vi "Draw Image to Picture (ARGB with Mask).vi"(7 "Image Draw Offset (Default 0,0)":T2, 8 "error in (no error)":errorcluster, 10 "Greyscale Mask in":T1, 11 "ARGB Image Source in":T3) -> (0 "error out":errorcluster, 3 "Picture":picture)   [LabVIEW 2020, in "image.lvlib"]
doc: "Draw an image to a LabVIEW Picture with Mask Data to allow for the output picture to be concatinated with other LabVIEW Picture Data."
uses:
  image.lvlib
  ARGB Image.ctl
  Image Draw Offset.ctl
  Greyscale Image.ctl
  8cd07b1b-062e-4fe4-9e87-2eb3dc89fe0e.vi
  <vilib>/Utility/error.llb/Error Cluster From Error Code.vi
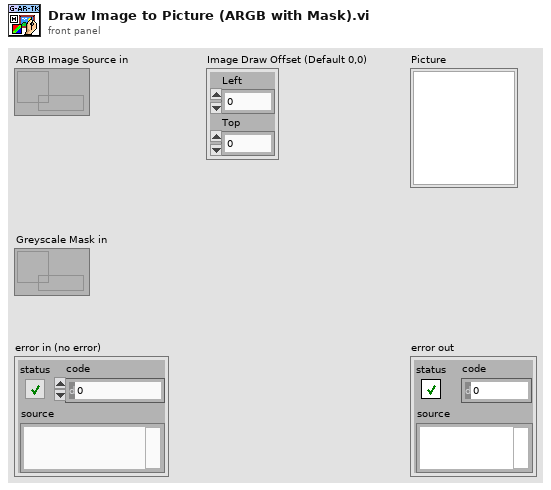
[diagram p1: front panel]
types:
  T1 = typedef "image.lvlib/Greyscale Image.ctl" = refnum<data-value>
  T2 = typedef "image.lvlib/Image Draw Offset.ctl" = cluster{"Left":i16, "Top":i16}
  T3 = typedef "image.lvlib/ARGB Image.ctl" = refnum<data-value>
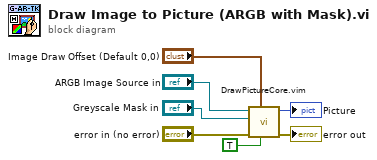
[diagram p0: block diagram]
diagram:
  n1 = call "DrawPictureCore.vim"("HasMask"=TRUE, "Image Draw Offset"="Image Draw Offset (Default 0,0)", "error in (no error)"="error in (no error)", "Image Mask"="Greyscale Mask in", "Image Src"="ARGB Image Source in") -> ("error out"=→"error out":errorcluster, "Picture"=→"Picture":picture)  [unwired: 5 in]
